vi "Prioritize Coin Placement.vi"(0 "Candidate Cells":i32[](array[numeric]), 1 "Board Array":T2[](array[typedef]), 5 "Moving to Opp. King's Neighbour?":bool, 7 "Move Index":i32, 9 "Parsed Board Info":T1, 11 "error in (no error)":errorcluster, 12 "Net Cell Gain":i32, 13 "Danger Free DT Cells":i32[](array[numeric])) -> (4 "Move Index":i32, 15 "error out":errorcluster)   [LabVIEW 2014]
uses:
  Typedefs/Board Cell.ctl
  Typedefs/Cell Occupancy.ctl
  Typedefs/Parsed Board.ctl
  <userlib>/_OpenG.lib/array/array.llb/Filter 1D Array with Scalar (I32)__ogtk.vi
  Dragon Tamers.lvlib
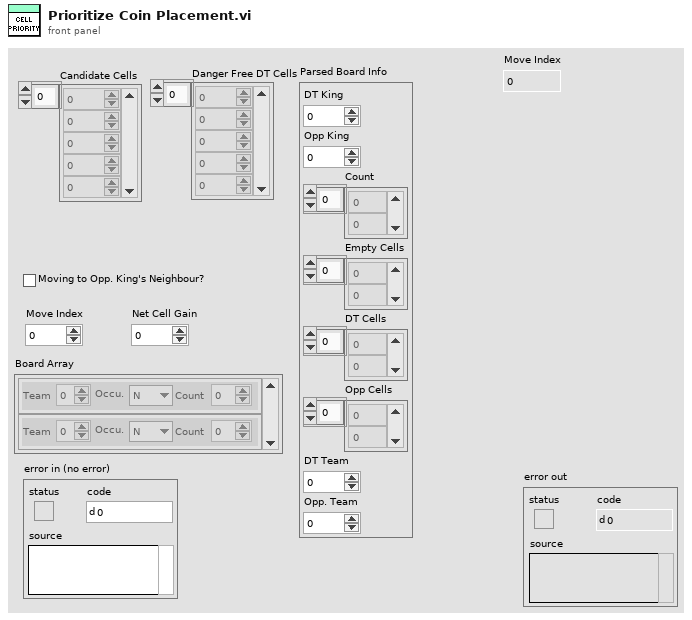
[diagram p1: front panel]
types:
  T1 = typedef "Dragon Tamers.lvlib/Parsed Board.ctl" = cluster{"DT King":i32, "Opp King":i32, "Count":i32[], "Empty Cells":i32[], "DT Cells":i32[], "Opp Cells":i32[], "DT Team":i32, "Opp. Team":i32}
  T2 = typedef "Dragon Tamers.lvlib/Board Cell.ctl" = cluster{"Team":i32, "Occu.":T3, "Count":i32}
  T3 = typedef "Dragon Tamers.lvlib/Cell Occupancy.ctl" = enum16{"N", "C", "K"}
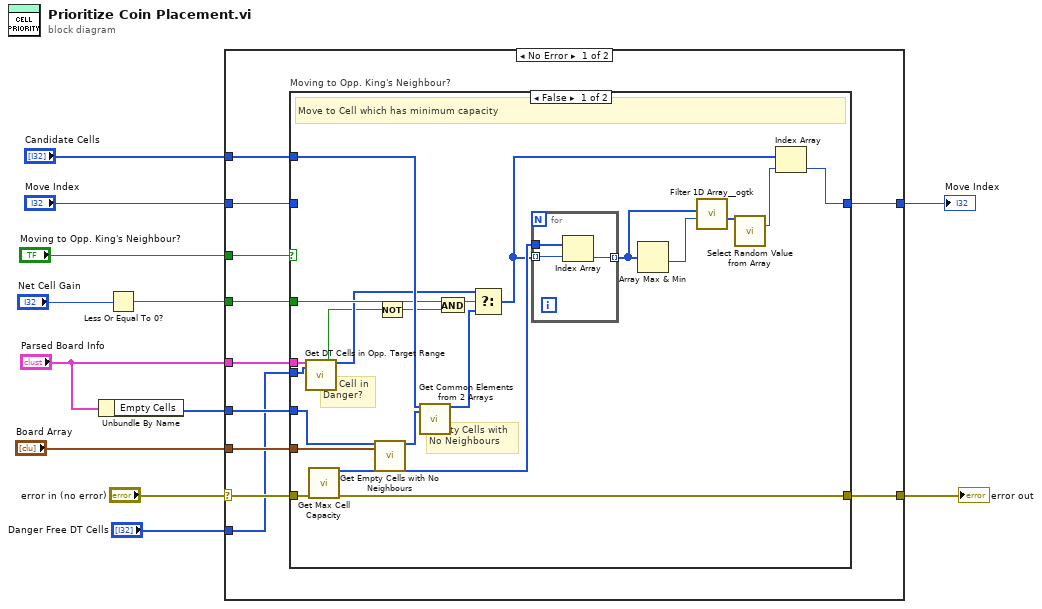
[diagram p0: block diagram]
diagram:
  n1 = Unbundle By Name("Parsed Board Info") -> ("Empty Cells"=w5:i32[])
  n2 = Less Or Equal To 0?(x="Net Cell Gain") -> (x <= 0?=w2:bool)
  n3 = case shown="No Error" "error in (no error)" {
    selector: "error in (no error)" -> [w18 w51]
    tunnel: [w19 w51] -> w11
    tunnel: "Moving to Opp. King's Neighbour?" -> [w23 _]
    tunnel: [w22 w50] -> w9
    tunnel: "Move Index" -> [w21 w50]
    tunnel: "Candidate Cells" -> [w20 _]
    tunnel: w5 -> [w17 _]
    tunnel: "Board Array" -> [w16 _]
    tunnel: "Parsed Board Info" -> [w15 _]
    tunnel: w2 -> [w14 _]
    tunnel: "Danger Free DT Cells" -> [w13 _]
    frame No Error {
      n4 = case "Moving to Opp. King's Neighbour?" shown="False" w23 {
        tunnel: [w41 w49] -> w22
        tunnel: w21 -> [_ w49]
        tunnel: w20 -> [w36 _]
        tunnel: [w43 w48] -> w19
        tunnel: w18 -> [w44 w48]
        tunnel: w17 -> [w35 _]
        tunnel: w16 -> [w34 _]
        tunnel: w15 -> [w32 _]
        tunnel: w14 -> [w30 _]
        tunnel: w13 -> [w31 _]
        frame False {
          # "Empty Cells with\nNo Neighbours"
          # "DT Cell in\nDanger?"
          # "Move to Cell which has minimum capacity"
          n5 = call "Get DT Cells in Opp. Target Range.vi"("Parsed Board Info"=w32, "Danger Free DT Cells"=w31) -> ("Empty?"=w25:bool, "Intended Array"=w29:i32[])  [unwired: 15 in, 1 out]
          n6 = call "Get Max Cell Capacity.vi"("error in (no error)"=w44) -> ("Max Capacity[]"=w42:i32[], "error out"=w43:errorcluster)  [unwired: 13 in]
          n7 = call "Get Empty Cells with No Neighbours.vi"("Empty Cells"=w35, "Board Array"=w34) -> ("Intended Array"=w33:i32[])  [unwired: 15 in, 2 out]
          n8 = Not(x=w25) -> (.not. x?=w24:bool)
          n9 = call "Get Common Elements from 2 Arrays.vi"("Array 1"=w36, "Array 2"=w33) -> ("Intended Array"=w28:i32[])  [unwired: 15 in, 2 out]
          n10 = And(x=w30, y=w24) -> (x .and. y?=w26:bool)
          n11 = Select(t=w29, s=w26, f=w28) -> (s? t:f=w27:i32[])
          n12 = for {
            tunnel: w27 -> [w47] mode=indexing
            tunnel: w42 -> [w46]
            tunnel: [w45] -> w39 mode=indexing
            n13 = Index Array(array=w46, index=w47) -> (element=w45:i32)
          }
          n14 = Array Max & Min(array=w39) -> (min value=w40:i32)  [unwired: 3 out]
          n15 = call-poly <userlib>:"Filter 1D Array__ogtk.vi"("items to filter"=w40, "array"=w39) -> ("filtered item indices"=w38:i32[])  [unwired: 4 in, 1 out]
          n16 = call "Select Random Value from Array.vi"("Array"=w38) -> ("Selected Value"=w37:i32)  [unwired: 11 in, 3 out]
          n17 = Index Array(array=w27, index=w37) -> (element=w41:i32)
        }
        frame True {
        }
      }
    }
    frame Error {
    }
  }
  "error out" <- w11
  "Move Index" <- w9
